vi "H5Pget_external.vi"(6 "error in (no error)":errorcluster, 8 "Index":u32, 9 "HDF5 Property Ref":T1) -> (0 "error out":errorcluster, 1 "Size":u64, 2 "Path":path, 3 "HDF5 Ref out":T1, 4 "Offset":i32)   [LabVIEW 2017]
doc: "Returns information about an external file."
uses:
  <vilib>/UPVI/lvhdf5/library.llb/HDF5 Ref.ctl
  <vilib>/UPVI/lvhdf5/hdf5.dll
panel:
  # "LVHDF5 Toolkit\nCopyright (c) 2005-2013 by Jason D. Sommerville\nCopyright (c) 2014 by UPVI, LLC.\n\nThis use and distribution of this file is governed by the terms found in \nLICENSE.txt distributed with this toolkit and installed at\n <user.lib>\\_lvhdf5\\LICENSE.txt"
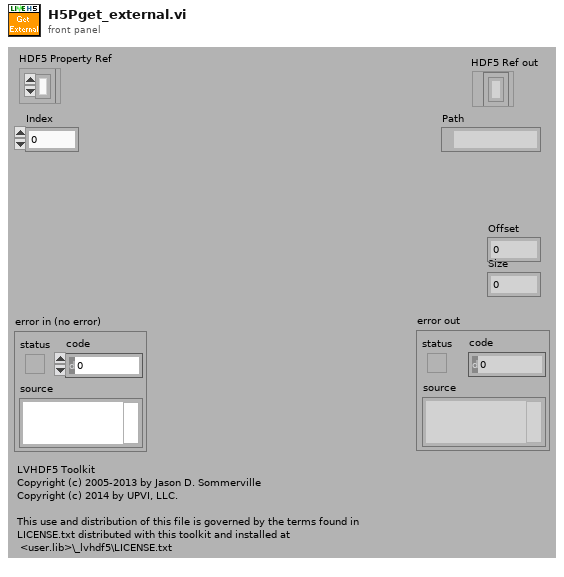
[diagram p1: front panel]
types:
  T1 = typedef "HDF5 Ref.ctl" = refnum<k1>
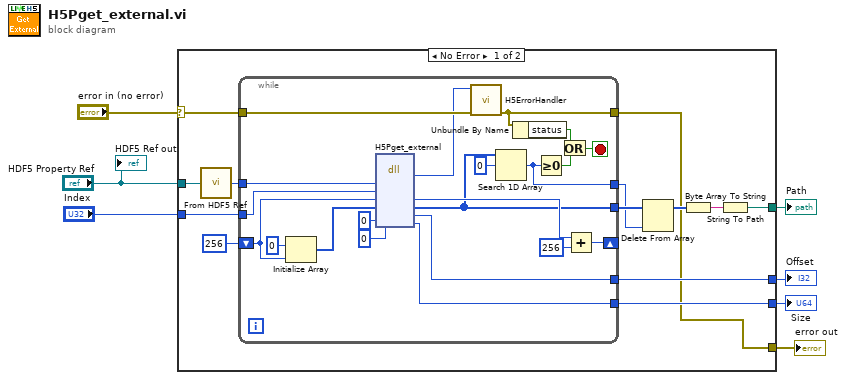
[diagram p0: block diagram]
diagram:
  n1 = case shown="No Error" "error in (no error)" {
    selector: "error in (no error)" -> [w20 w42]
    tunnel: [w8 w42] -> w6
    tunnel: "HDF5 Property Ref" -> [w19 _]
    tunnel: "Index" -> [w17 _]
    tunnel: [w11 _] -> w1
    tunnel: [w10 _] -> w2
    tunnel: [w9 _] -> w3
    frame No Error {
      n2 = call <vilib>:"From HDF5 Ref.vi"("HDF5 Ref"=w19) -> ("I32"=w18:i32)
      n3 = while {
        tunnel: w20 -> [w41]
        tunnel: [w25] -> w8
        tunnel: w18 -> [w40]
        shift-right: [w30] -> _
        shift-left: 256 -> [w33]
        tunnel: w17 -> [w38]
        tunnel: [w31] -> w10
        tunnel: [w26] -> w15
        tunnel: [w21] -> w14
        tunnel: [w32] -> w9
        stop <- w22 stop-if-true
        n4 = Initialize Array(u8 0 ("element"), w33) -> (w34:u8[])
        n5 = dll-call lib="C:/Program Files/National Instruments/LabVIEW 2017/vi.lib/UPVI/lvhdf5/hdf5.dll" fn="H5Pget_external"("plist_id"=w40, "idx"=w38, "name_size"=w33, "name"=w34, "offset"=0, "size"=u64 0) -> ("return type"=w39:i32, "name_size"=w28:u32, "name"=w26:u8[], "offset"=w31:i32, "size"=w32:u64)  [unwired: 5 in, 2 out]
        n6 = call <vilib>:"H5ErrorHandler.vi"("error in (no error)"=w41, "herr_t"=w39) -> ("error out"=w25:errorcluster)  [unwired: 3 in, 4 out]
        n7 = Search 1D Array(1D array=w26, element=u8 0) -> (index of element=w21:i32)  [unwired: 1 in]
        n8 = Unbundle By Name(w25) -> ("status"=w24:bool)
        n9 = Greater Or Equal To 0?(x=w21) -> (x >= 0?=w23:bool)
        n10 = Or(x=w24, y=w23) -> (x .or. y?=w22:bool)
        n11 = Add(x=w28, y=u32 256) -> (x+y=w30:u32)
      }
      n12 = Delete From Array(array=w15, index=w14) -> (array with subset deleted=w13:u8[])  [unwired: 1 in, 1 out]
      n13 = Byte Array To String(unsigned byte array=w13) -> (string=w12:string)
      n14 = String To Path(string=w12) -> (path=w11:path)
    }
    frame Error {
    }
  }
  "error out" <- w6
  "Size" <- w3
  "Offset" <- w2
  "Path" <- w1
  "HDF5 Ref out" <- "HDF5 Property Ref"
